vi "SSL Detection Robot Referee.vi"(8 "error in":errorcluster, 9 "team_info_array_in":u8[](array[numeric]) format="%02x") -> (0 "error out":errorcluster, 1 "Length-delimited":u8[](array[numeric]) format="%02x", 3 "team info out":T1)   [LabVIEW 2023]
uses:
  SSL Referee Team Info.ctl
  Varint Decoder uint32.vi
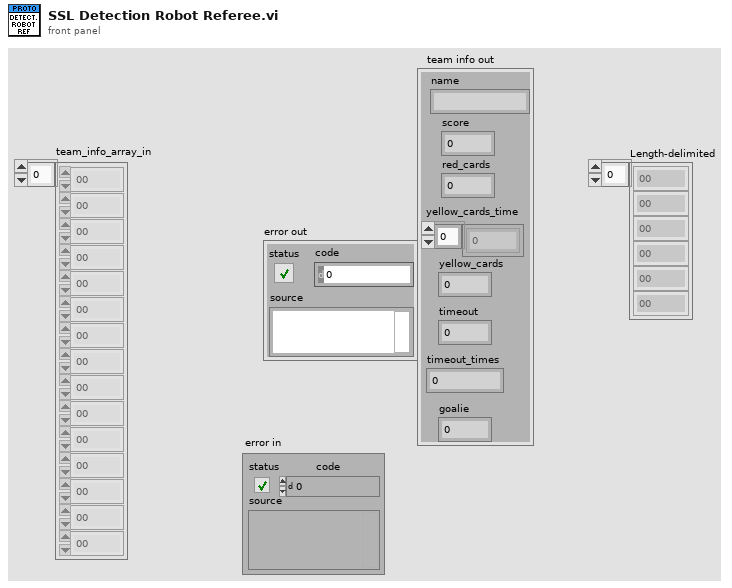
[diagram p1: front panel]
types:
  T1 = typedef "SSL Referee Team Info.ctl" = cluster{"name":string, "score":u32, "red_cards":u32, "yellow_cards_time":u32[], "yellow_cards":u32, "timeout":u32, "timeout_times":u32, "goalie":u32}
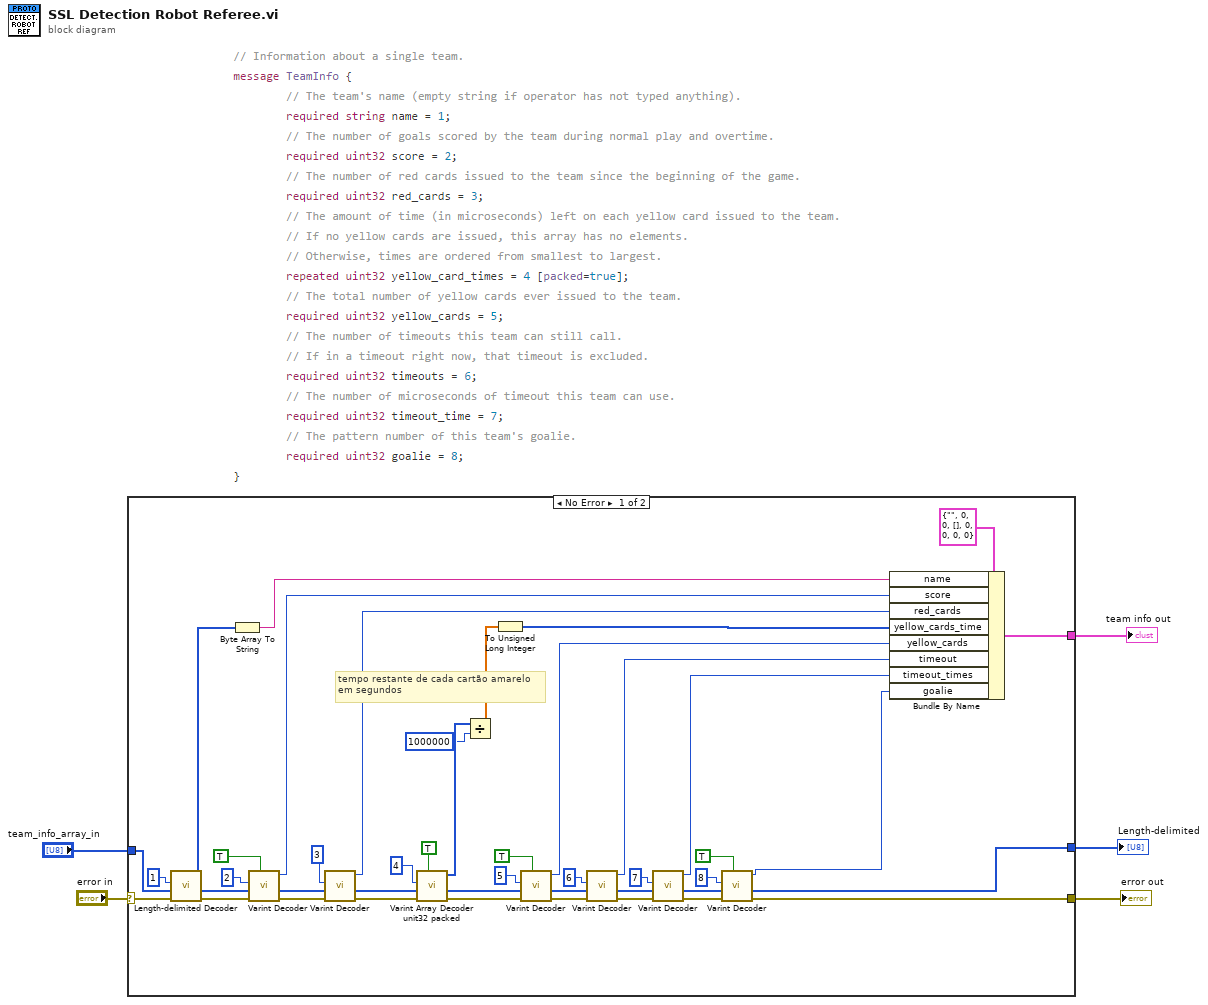
[diagram p0: block diagram]
diagram:
  n1 = case shown="No Error" "error in" {
    selector: "error in" -> [w48 w51]
    tunnel: [w35 w51] -> w4
    tunnel: [w36 w50] -> w3
    tunnel: "team_info_array_in" -> [w27 w50]
    tunnel: [w16 _] -> w1
    frame No Error {
      # "tempo restante de cada cartão amarelo\nem segundos"
      n2 = call "Length-delimited Decoder.vi"("error in (no error)"=w48, "Array"=w27, "Key"=1) -> ("error out"=w47:errorcluster, "array w/ subset deleted"=w26:u8[], "Length-delimited"=w25:u8[])  [unwired: 5 in, 1 out]
      n3 = Byte Array To String(unsigned byte array=w25) -> (string=w23:string)
      n4 = call-poly "Varint Decoder.vi"("Optional"=TRUE, "error in (no error)"=w47, "Array"=w26, "Key"=2) -> ("error out"=w46:errorcluster, "array w/ subset deleted"=w29:u8[], "Varint"=w22:u32)  [unwired: 4 in, 1 out]
      n5 = call-poly "Varint Decoder.vi"("error in (no error)"=w46, "Array"=w29, "Key"=3) -> ("error out"=w8:errorcluster, "array w/ subset deleted"=w15:u8[], "Varint"=w21:u32)  [unwired: 5 in, 1 out]
      n6 = call "Varint Array Decoder unit32 packed.vi"("Optional"=TRUE, "error in"=w8, "array in"=w15, "Key"=4) -> ("error out"=w7:errorcluster, "array w/ subset deleted"=w14:u8[], "varint_array"=w12:u32[])  [unwired: 5 in]
      n7 = Divide(x=w12, y=1000000) -> (x/y=w9:dbl[])
      n8 = To Unsigned Long Integer(number=w9) -> (unsigned 32bit integer=w10:u32[])
      n9 = call-poly "Varint Decoder.vi"("Optional"=TRUE, "error in (no error)"=w7, "Array"=w14, "Key"=5) -> ("error out"=w41:errorcluster, "array w/ subset deleted"=w31:u8[], "Varint"=w20:u32)  [unwired: 4 in, 1 out]
      n10 = call-poly "Varint Decoder.vi"("error in (no error)"=w41, "Array"=w31, "Key"=6) -> ("error out"=w39:errorcluster, "array w/ subset deleted"=w32:u8[], "Varint"=w19:u32)  [unwired: 5 in, 1 out]
      n11 = call-poly "Varint Decoder.vi"("error in (no error)"=w39, "Array"=w32, "Key"=7) -> ("error out"=w37:errorcluster, "array w/ subset deleted"=w33:u8[], "Varint"=w18:u32)  [unwired: 5 in, 1 out]
      n12 = call-poly "Varint Decoder.vi"("Optional"=TRUE, "error in (no error)"=w37, "Array"=w33, "Key"=8) -> ("error out"=w35:errorcluster, "array w/ subset deleted"=w36:u8[], "Varint"=w17:u32)  [unwired: 4 in, 1 out]
      n13 = Bundle By Name(cluster=T1 {"name"="", "score"=0, "red_cards"=0, "yellow_cards_time"=[], "yellow_cards"=0, "timeout"=0, "timeout_times"=0, "goalie"=0} ("team info"), "name"=w23, "score"=w22, "red_cards"=w21, "yellow_cards_time"=w10, "yellow_cards"=w20, "timeout"=w19, "timeout_times"=w18, "goalie"=w17) -> (w16:T1)
    }
    frame Error {
    }
  }
  "error out" <- w4
  "Length-delimited" <- w3
  "team info out" <- w1
